vi "EuniceF_Lab5Labview.vi"() -> ()   [LabVIEW 2025]
panel:
  out "AtoD":i16
  in  "stop":bool
  out "Boolean 2":bool
  out "Boolean":bool
  out "Height, cm":dbl(slide) scale=0.0..10.0
  out "P, in(H2O)":dbl(slide) scale=0.0..10.0
  out "Isens,mA":dbl(slide) scale=0.0..10.0
  out "Vin,V":dbl(slide) scale=0.0..10.0
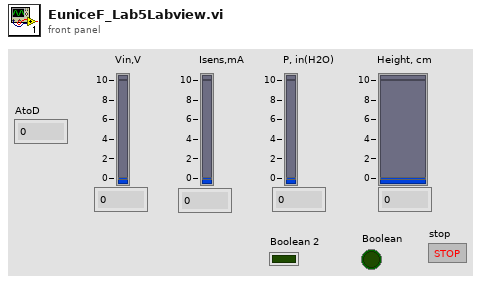
[diagram p1: front panel]
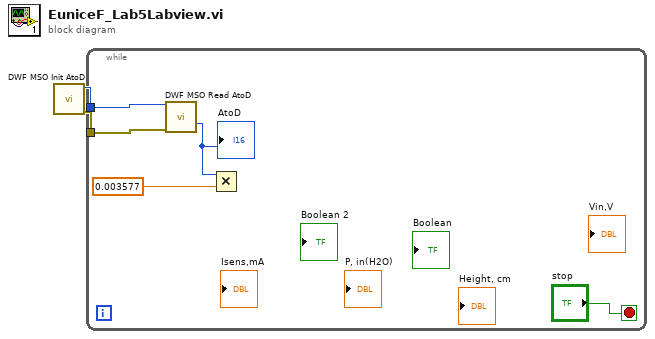
[diagram p0: block diagram]
diagram:
  n1 = call "DWF MSO Init AtoD.vi"() -> ("Error Out"=w1:errorcluster, "Instrument Handle Out"=w2:i32)  [unwired: 10 in]
  n2 = while {
    tunnel: w2 -> [w7]
    tunnel: w1 -> [w6]
    stop <- "stop" stop-if-true
    n3 = call "DWF MSO Read AtoD.vi"("Instrument Handle In AtoD"=w7, "Error In"=w6) -> ("AtoD"=w3:i16)  [unwired: 12 in, 1 out]
    "AtoD" <- w3
    n4 = Multiply(x=w3, y=0.003577) -> ()  [unwired: 1 out]
  }
